vi "RS232 Read Integer Editor.vi"() -> ()   [LabVIEW 2013]
uses:
  <vilib>/Utility/miscctls.llb/LVBoundsTypeDef.ctl
  CRYCustom and Run Seq.llb/CRYCustom Cluster.ctl
  CRYCustom and Run Seq.llb/CRYProject Editor Global.vi
  CRYCustom and Run Seq.llb/CRYStepSetup Global.vi
  CRYCustom and Run Seq.llb/CRYMainGlobal.vi
  CRYCustom and Run Seq.llb/CRYMain Sub Window Global.vi
panel:
  out "Custom":string
  out "Custom Bk":string
  in  "AddStep":bool
  in  "Add Lib":bool
  in  "stop":bool
  in  "Load Test":bool
  out "EndFlag":bool
  out "Proper VI No":i32
  in  "Save As":bool
  in  "Load":bool
  in  "Revert":bool
  out "VIMiniumBound":T1
  in  "Board Tab":enum32{"Page 1"}(tab) caption="Control Tab"
  in  "Cancel":bool caption="Apply"
  in  "OK":bool caption="Apply"
  in  "Sub Board Tab":enum32{"Setting", "Help"}(tab)
  out "Comment":bool
  in  "Unit":string
  in  "Byte":i32
  in  "Curve Name":string caption="Name"
  in  "Select COM Port":i32(ring) items=["COM1", "COM2", "COM3", "COM4", "COM5", "COM6", "COM7", "COM8", "COM9", "COM10", "COM11", "COM12", "COM13", "COM14", "COM15", "COM16", "COM17", "COM18", "COM19", "COM20"]
  out "Reminder":bool
  in  "Help":string
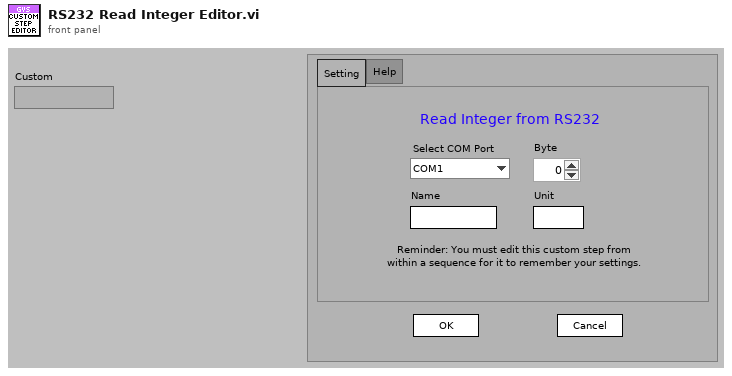
[diagram p1: front panel]
types:
  T1 = typedef "LVBoundsTypeDef.ctl" = cluster{"Width":u32, "Height":u32}
  T2 = cluster{"Type":u16, "Select COM Port":i32, "Byte":i32, "Unit":string, "Curve Name":string}
  T3 = typedef "CRYStep.ctl" = cluster{"No.VI":i32, "Category":string, "StepName":string, "Seq setup flattened":string, "Comment":string, "Steps config.":bool[], "Jump config":i32[], "Start":dbl, "Increment":dbl, "Name":string, "Unit":string, "Y data":u16, "Y prefix":string, "Y dB ref":dbl, "Y unit":string, "Repeat State Array":cluster{"Start":dbl, "Increment":dbl, "Count":i32, "Num":i32}[]}
  T4 = typedef "CRYCustom Cluster.ctl" = cluster{"Help":string, "Flatten Data":string}
  T5 = cluster{"Load Test":bool, "Add Lib":bool, "OK":bool, "Cancel":bool}
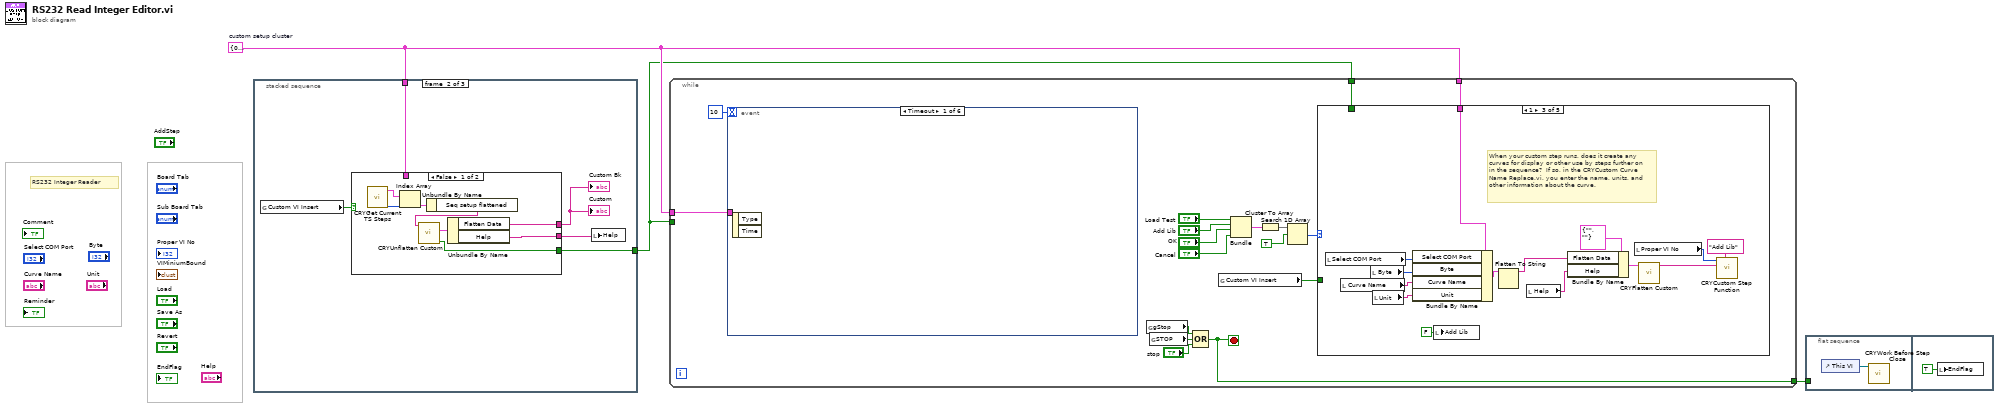
[diagram p0: block diagram]
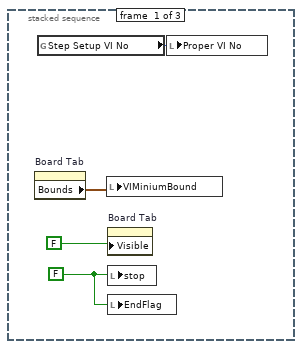
[diagram p2: hidden frame]
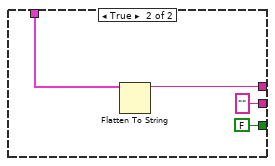
[diagram p3: hidden frame]
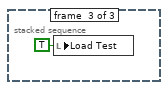
[diagram p4: hidden frame]
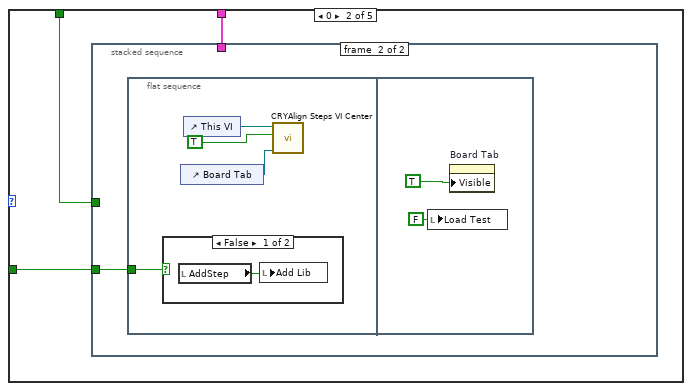
[diagram p6: hidden frame]
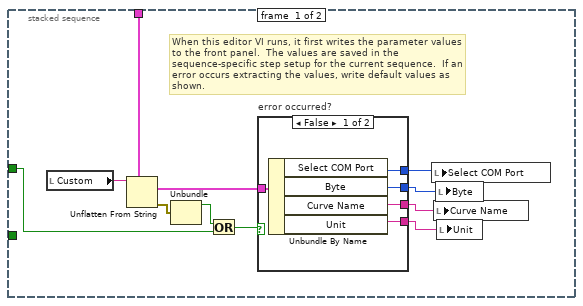
[diagram p7: hidden frame]
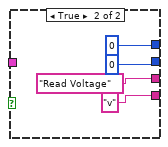
[diagram p8: hidden frame]
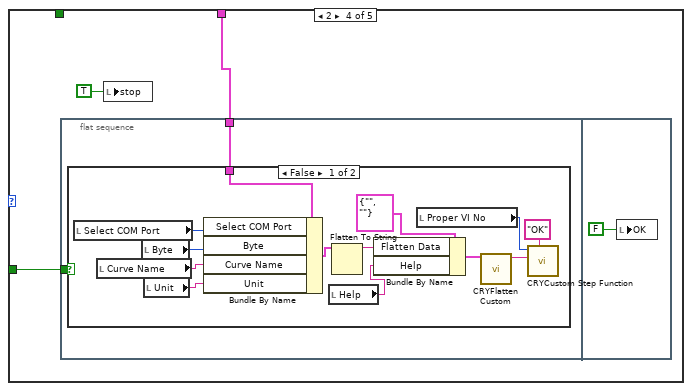
[diagram p10: hidden frame]
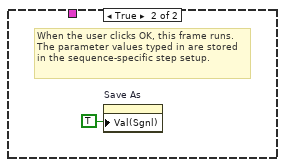
[diagram p11: hidden frame]
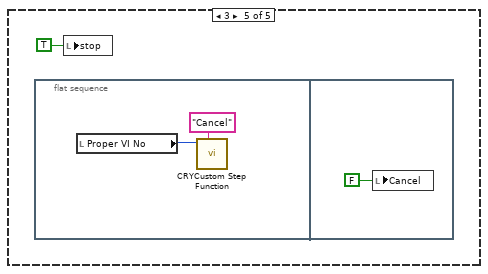
[diagram p12: hidden frame]
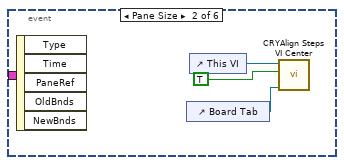
[diagram p13: hidden frame]
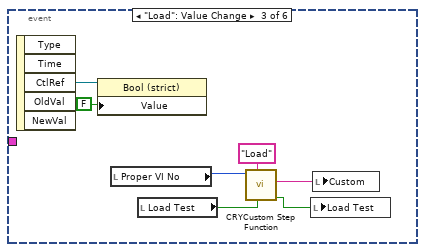
[diagram p14: hidden frame]
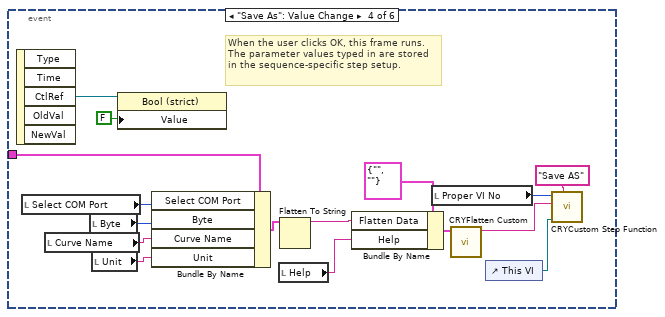
[diagram p15: hidden frame]
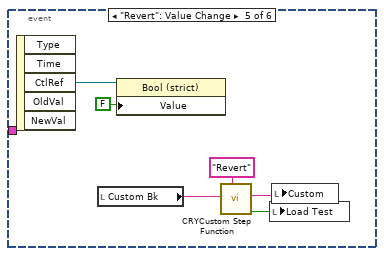
[diagram p16: hidden frame]
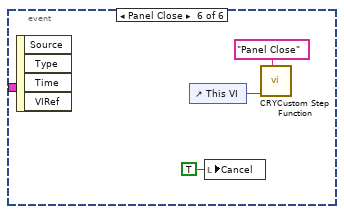
[diagram p17: hidden frame]
diagram:
  w2 = T2 {"Type"=0, "Select COM Port"=0, "Byte"=0, "Unit"="v", "Curve Name"="Read Voltage"}  # custom setup cluster
  # "RS232 Integer Reader"
  n1 = stacked-sequence {
    tunnel: w2 -> [_ w11 _]
    tunnel: [_ w10 _] -> w1
    frame #0 {
      w4 = FALSE ("stop")
      n2 = property on="Board Tab" class="TabCtl (strict)"() -> ("Bounds"=w7:T1)  [unwired: 2 in, 2 out]
      n3 = global read "CRYProject Editor Global.vi" "Step Setup VI No"() -> (w5:i32)
      n4 = local write "VIMiniumBound"(w7) -> ()
      n5 = property on="Board Tab" class="TabCtl (strict)"("Visible"=FALSE ("Load Test")) -> ()  [unwired: 2 in, 2 out]
      n6 = local write "stop"(w4) -> ()
      n7 = local write "EndFlag"(w4) -> ()
      n8 = local write "Proper VI No"(w5) -> ()
    }
    frame #1 {
      n9 = global read "CRYStepSetup Global.vi" "Custom VI Insert"() -> (w12:bool)
      n10 = case shown="False" w12 {
        tunnel: [w14 w23] -> w9
        tunnel: w11 -> [_ w24]
        tunnel: [w16 FALSE ("Error?")] -> w10
        tunnel: [w13 "" ("Help")] -> w8
        frame False {
          n11 = call "CRYGet Current TS Steps.vi"() -> ("SelectStepNumber in Tree"=w18:i32, "Steps"=w19:T3[])  [unwired: 7 in, 3 out]
          n12 = Index Array(array=w19, index=w18) -> (element=w20:T3)
          n13 = Unbundle By Name(w20) -> ("Seq setup flattened"=w15:string)
          n14 = call "CRYUnflatten Custom.vi"("Unflatten Custom"=w15) -> ("Error?"=w16:bool, "Custom"=w17:T4)  [unwired: 8 in, 1 out]
          n15 = Unbundle By Name(w17) -> ("Flatten Data"=w14:string, "Help"=w13:string)
        }
        frame True {
          n16 = Flatten To String(anything=w24) -> (data string=w23:string)  [unwired: 1 in, 4 out]
        }
      }
      "Custom" <- w9
      "Custom Bk" <- w9
      n17 = local write "Help"(w8) -> ()
    }
    frame #2 {
      n18 = local write "Load Test"(TRUE ("Load Test")) -> ()
    }
  }
  n19 = while {
    tunnel: [w33] -> w3
    tunnel: w2 -> [w28]
    tunnel: w2 -> [w27]
    tunnel: w1 -> [w26]
    tunnel: w1 -> [_]
    stop <- w33 stop-if-true
    n20 = event shown="[0] Timeout" {
      selector: _ -> [_ _ _ _ _ _]
      dyn-events: _ -> [_ _ _ _ _ _]
      timeout: 10 -> [_ _ _ _ _ _]
      tunnel: w27 -> [_ _ _ w130 _ _]
      event Timeout {
        n21 = event-data() -> ()  [unwired: 1 in, 2 out]
      }
      event Pane Size {
        n22 = event-data() -> ()  [unwired: 1 in, 5 out]
        n23 = control-ref of="Board Tab"() -> (w112:refnum<vi>)
        n24 = control-ref of="This VI"() -> (w113:refnum<vi>)
        n25 = call "CRYAlign Steps VI Center.vi"("Tab2"=w112, "Input/Output"=TRUE ("Preview"), "VIRef"=w113) -> ()  [unwired: 1 in, 8 out]
      }
      event "Load": Value Change {
        n26 = event-data() -> ("CtlRef"=w120:refnum<vi>)  [unwired: 1 in, 4 out]
        n27 = property class="Bool (strict)"(reference=w120, "Value"=FALSE) -> ()  [unwired: 1 in, 2 out]
        n28 = local read "Proper VI No"() -> (w115:i32)
        n29 = local read "Load Test"() -> (w116:bool)
        n30 = call "CRYCustom Step Function.vi"("bData"=w116, "sAction"="Load" ("Action"), "nData"=w115) -> ("bData Out"=w117:bool, "sData Out"=w118:string)  [unwired: 7 in]
        n31 = local write "Load Test"(w117) -> ()
        n32 = local write "Custom"(w118) -> ()
      }
      event "Save As": Value Change {
        # "When the user clicks OK, this frame runs.  The parameter values typed in are stored in the sequence-specific step setup."
        n33 = event-data() -> ("CtlRef"=w136:refnum<vi>)  [unwired: 1 in, 4 out]
        n34 = local read "Select COM Port"() -> (w132:i32)
        n35 = local read "Curve Name"() -> (w134:string)
        n36 = local read "Byte"() -> (w133:i32)
        n37 = local read "Unit"() -> (w135:string)
        n38 = property class="Bool (strict)"(reference=w136, "Value"=FALSE) -> ()  [unwired: 1 in, 2 out]
        n39 = Bundle By Name(cluster=w130, "Select COM Port"=w132, "Byte"=w133, "Curve Name"=w134, "Unit"=w135) -> (w131:T2)
        n40 = local read "Help"() -> (w126:string)
        n41 = Flatten To String(anything=w131) -> (data string=w129:string)  [unwired: 1 in, 4 out]
        n42 = Bundle By Name(cluster=T4 {"Help"="", "Flatten Data"=""} ("Custom"), "Flatten Data"=w129, "Help"=w126) -> (w128:T4)
        n43 = local read "Proper VI No"() -> (w123:i32)
        n44 = call "CRYFlatten Custom.vi"("Custom"=w128) -> ("Flatten Custom String"=w122:string)  [unwired: 10 in]
        n45 = control-ref of="This VI"() -> (w124:refnum<vi>)
        n46 = call "CRYCustom Step Function.vi"("sAction"="Save AS" ("Action"), "VI Ref"=w124, "sData"=w122, "nData"=w123) -> ()  [unwired: 6 in, 2 out]
      }
      event "Revert": Value Change {
        n47 = event-data() -> ("CtlRef"=w143:refnum<vi>)  [unwired: 1 in, 4 out]
        n48 = local read "Custom Bk"() -> (w139:string)
        n49 = property class="Bool (strict)"(reference=w143, "Value"=FALSE) -> ()  [unwired: 1 in, 2 out]
        n50 = call "CRYCustom Step Function.vi"("sAction"="Revert" ("Action"), "sData"=w139) -> ("bData Out"=w140:bool, "sData Out"=w138:string)  [unwired: 8 in]
        n51 = local write "Load Test"(w140) -> ()
        n52 = local write "Custom"(w138) -> ()
      }
      event Panel Close {
        n53 = event-data() -> ()  [unwired: 1 in, 4 out]
        n54 = control-ref of="This VI"() -> (w144:refnum<vi>)
        n55 = local write "Cancel"(TRUE ("Cancel")) -> ()
        n56 = call "CRYCustom Step Function.vi"("sAction"="Panel Close" ("Action"), "VI Ref"=w144) -> ()  [unwired: 8 in, 2 out]
      }
    }
    n57 = global read "CRYMain Sub Window Global.vi" "gStop"() -> (w36:bool)
    n58 = global read "CRYMainGlobal.vi" "STOP"() -> (w34:bool)
    n59 = Compound Arithmetic op=OR(w36, w34, "stop") -> (w33:bool)
    n60 = global read "CRYStepSetup Global.vi" "Custom VI Insert"() -> (w29:bool)
    n61 = Bundle("Load Test"="Load Test", "Add Lib"="Add Lib", "OK"="OK", "Cancel"="Cancel") -> (w40:T5)  [unwired: 1 out]
    n62 = Cluster To Array(cluster=w40) -> (array=w39:bool[])
    n63 = Search 1D Array(1D array=w39, element=TRUE) -> (index of element=w37:i32)  [unwired: 1 out]
    n64 = case shown="1" w37 {
      tunnel: w29 -> [_ w45 _ w89 _]
      tunnel: w28 -> [_ w44 w81 w88 _]
      tunnel: w26 -> [_ w43 _ _ _]
      frame Default {
      }
      frame 0 {
        n65 = stacked-sequence {
          tunnel: w45 -> [_ w66]
          tunnel: w44 -> [w52 _]
          tunnel: w43 -> [w46 _]
          frame #0 {
            # "When this editor VI runs, it first writes the parameter values to the front panel.  The values are saved in the sequence-specific step setup for the current sequence.  If an error occurs extracting the values, write default values as shown."
            n66 = local read "Custom"() -> (w47:string)
            n67 = Unflatten From String(type=w52, binary string=w47) -> (value=w55:T2, error out=w56:errorcluster)  [unwired: 1 in, 3 out]
            n68 = Unbundle(w56) -> ("status"=w53:bool)  [unwired: 2 out]
            n69 = Or(x=w53, y=w46) -> (x .or. y?=w54:bool)
            n70 = case "error occurred?" shown="False" w54 {
              tunnel: w55 -> [w61 _]
              tunnel: [w60 0 ("Select COM Port")] -> w51
              tunnel: [w59 0 ("Byte")] -> w50
              tunnel: [w58 "Read Voltage" ("Curve Name")] -> w49
              tunnel: [w57 "v" ("Unit")] -> w48
              frame False {
                n71 = Unbundle By Name(w61) -> ("Select COM Port"=w60:i32, "Byte"=w59:i32, "Curve Name"=w58:string, "Unit"=w57:string)
              }
              frame True {
              }
            }
            n72 = local write "Select COM Port"(w51) -> ()
            n73 = local write "Curve Name"(w49) -> ()
            n74 = local write "Byte"(w50) -> ()
            n75 = local write "Unit"(w48) -> ()
          }
          frame #1 {
            n76 = flat-sequence {
              tunnel: w66 -> [w67]
              frame #0 {
                n77 = case shown="False" w67 {
                  frame False {
                    n78 = local read "AddStep"() -> (w71:bool)
                    n79 = local write "Add Lib"(w71) -> ()
                  }
                  frame True {
                  }
                }
                n80 = control-ref of="Board Tab"() -> (w68:refnum<vi>)
                n81 = control-ref of="This VI"() -> (w69:refnum<vi>)
                n82 = call "CRYAlign Steps VI Center.vi"("Tab2"=w68, "Input/Output"=TRUE ("Preview"), "VIRef"=w69) -> ()  [unwired: 1 in, 8 out]
              }
              frame #1 {
                n83 = local write "Load Test"(FALSE ("Load Test")) -> ()
                n84 = property on="Board Tab" class="TabCtl (strict)"("Visible"=TRUE ("Load Test")) -> ()  [unwired: 2 in, 2 out]
              }
            }
          }
        }
      }
      frame 1 {
        # "When your custom step runs, does it create any curves for display or other use by steps further on in the sequence?  If so, in the CRYCustom Curve Name Replace.vi, you enter the name, units, and other information about the curve."
        n85 = local read "Select COM Port"() -> (w83:i32)
        n86 = local read "Curve Name"() -> (w85:string)
        n87 = local read "Byte"() -> (w84:i32)
        n88 = local read "Unit"() -> (w86:string)
        n89 = Bundle By Name(cluster=w81, "Select COM Port"=w83, "Byte"=w84, "Curve Name"=w85, "Unit"=w86) -> (w82:T2)
        n90 = local write "Add Lib"(FALSE ("Add Lib")) -> ()
        n91 = Flatten To String(anything=w82) -> (data string=w78:string)  [unwired: 1 in, 4 out]
        n92 = local read "Help"() -> (w77:string)
        n93 = Bundle By Name(cluster=T4 {"Help"="", "Flatten Data"=""} ("Custom"), "Flatten Data"=w78, "Help"=w77) -> (w79:T4)
        n94 = local read "Proper VI No"() -> (w74:i32)
        n95 = call "CRYFlatten Custom.vi"("Custom"=w79) -> ("Flatten Custom String"=w75:string)  [unwired: 10 in]
        n96 = call "CRYCustom Step Function.vi"("sAction"="Add Lib" ("Action"), "sData"=w75, "nData"=w74) -> ()  [unwired: 7 in, 2 out]
      }
      frame 2 {
        n97 = flat-sequence {
          tunnel: w89 -> [w92]
          tunnel: w88 -> [w91]
          frame #0 {
            n98 = case shown="False" w92 {
              tunnel: w91 -> [w105 _]
              frame False {
                n99 = local read "Select COM Port"() -> (w103:i32)
                n100 = local read "Curve Name"() -> (w101:string)
                n101 = local read "Byte"() -> (w102:i32)
                n102 = local read "Unit"() -> (w100:string)
                n103 = Bundle By Name(cluster=w105, "Select COM Port"=w103, "Byte"=w102, "Curve Name"=w101, "Unit"=w100) -> (w104:T2)
                n104 = local read "Help"() -> (w96:string)
                n105 = Flatten To String(anything=w104) -> (data string=w98:string)  [unwired: 1 in, 4 out]
                n106 = Bundle By Name(cluster=T4 {"Help"="", "Flatten Data"=""} ("Custom"), "Flatten Data"=w98, "Help"=w96) -> (w97:T4)
                n107 = local read "Proper VI No"() -> (w94:i32)
                n108 = call "CRYFlatten Custom.vi"("Custom"=w97) -> ("Flatten Custom String"=w93:string)  [unwired: 10 in]
                n109 = call "CRYCustom Step Function.vi"("sAction"="OK" ("Action"), "sData"=w93, "nData"=w94) -> ()  [unwired: 7 in, 2 out]
              }
              frame True {
                # "When the user clicks OK, this frame runs.  The parameter values typed in are stored in the sequence-specific step setup."
                n110 = property on="Save As" class="Bool (strict)"("Val(Sgnl)"=TRUE ("Value (Signaling)")) -> ()  [unwired: 2 in, 2 out]
              }
            }
          }
          frame #1 {
            n111 = local write "OK"(FALSE ("OK")) -> ()
          }
        }
        n112 = local write "stop"(TRUE ("stop")) -> ()
      }
      frame 3 {
        n113 = flat-sequence {
          frame #0 {
            n114 = local read "Proper VI No"() -> (w109:i32)
            n115 = call "CRYCustom Step Function.vi"("sAction"="Cancel" ("Action"), "nData"=w109) -> ()  [unwired: 8 in, 2 out]
          }
          frame #1 {
            n116 = local write "Cancel"(FALSE ("Cancel")) -> ()
          }
        }
        n117 = local write "stop"(TRUE ("stop")) -> ()
      }
    }
  }
  n118 = flat-sequence {
    tunnel: w3 -> [_]
    frame #0 {
      n119 = control-ref of="This VI"() -> (w147:refnum<vi>)
      n120 = call "CRYWork Before Step Close.vi"("StepVI Ref"=w147) -> ()  [unwired: 11 in]
    }
    frame #1 {
      n121 = local write "EndFlag"(TRUE ("EndFlag")) -> ()
    }
  }
